vi "SessionManagerSimulator.vi"() -> ()   [LabVIEW 2014]
uses:
  TimeStamper/TimeStamper.lvclass
panel:
  out "error out":errorcluster
  in  "Experimenter":string(combo)="Unselected"
  out "Session Path":path
  in  "stop":bool
  in  "Subject":string(combo)="Testing"
  in  "Counter Card":tag="Dev1"
  in  "Sample Lines":tag[](array[tag])=["/Dev3/ai/StartTrigger", "/Dev1/PXI_Trig4", "/4498_1/ai/StartTrigger"]
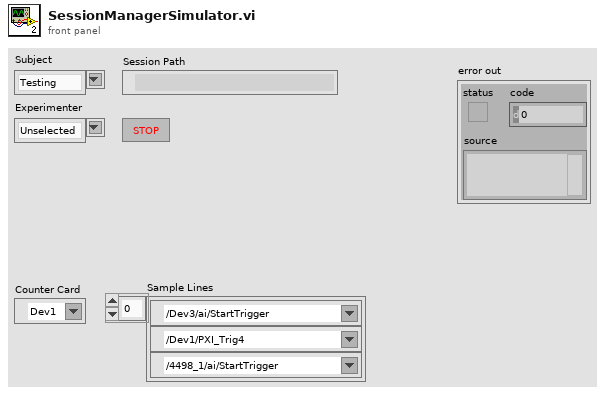
[diagram p1: front panel]
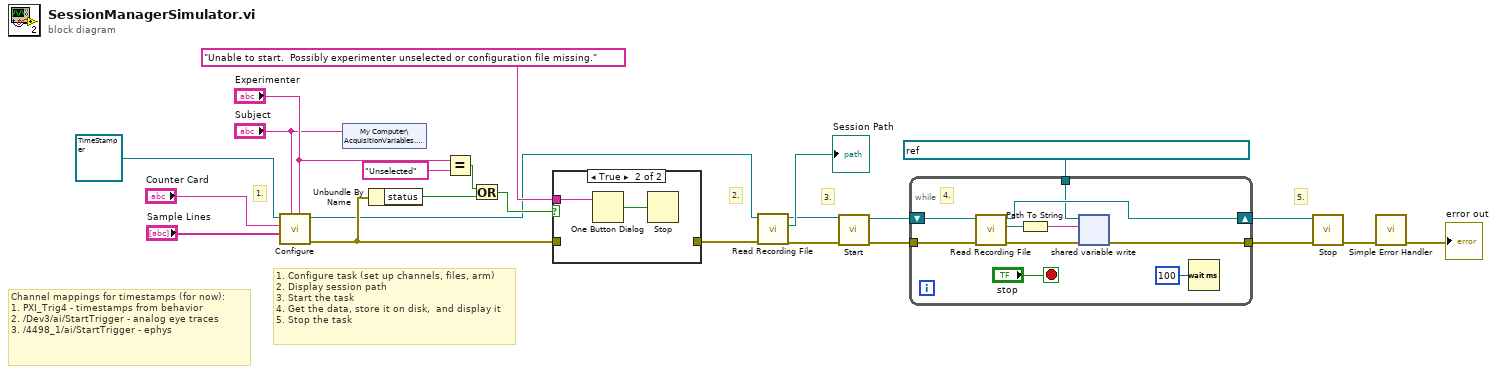
[diagram p0: block diagram]
diagram:
  # "Channel mappings for timestamps (for now):\n1. PXI_Trig4 - timestamps from behavior\n2. /Dev3/ai/StartTrigger - analog eye traces\n3. /4498_1/ai/StartTrigger - ephys"
  # "1. Configure task (set up channels, files, arm)\n2. Display session path\n3. Start the task\n4. Get the data, store it on disk,  and display it\n5. Stop the task"
  # "2."
  # "5."
  # "3."
  # "1."
  n1 = call-dynamic "Configure.vi"("Experimenter"="Experimenter", "Subject"="Subject", "Sample Lines"="Sample Lines", "DAQmx Device Name"="Counter Card", "TimeStamper in"=refnum<class "TimeStamper.lvclass"> refnum ("TimeStamper.lvclass")) -> ("error out"=w9:errorcluster, "TimeStamper out"=w8:refnum<class "TimeStamper.lvclass">)  [unwired: 5 in]
  n2 = shared-variable "My Computer\\AcquisitionVariables.lvlib\\Subject"("Subject") -> ()  [unwired: 1 in, 1 out]
  n3 = Unbundle By Name(w9) -> ("status"=w10:bool)
  n4 = Equal?(x="Experimenter", y="Unselected") -> (x = y?=w16:bool)
  n5 = Or(x=w16, y=w10) -> (x .or. y?=w15:bool)
  n6 = case shown="True" w15 {
    tunnel: "Unable to start.  Possibly experimenter unselected or configuration file missing." -> [_ w26]
    tunnel: w9 -> [w24 _]
    tunnel: [w24 _] -> w7
    frame False {
    }
    frame True {
      n7 = One Button Dialog(message=w26) -> (true=w25:bool)  [unwired: 1 in]
      n8 = Stop(stop? (T)=w25) -> ()
    }
  }
  n9 = call-dynamic "Read Recording File.vi"("error in (no error)"=w7, "AcquistionObject in"=w8) -> ("error out"=w4:errorcluster, "Recording File"=→"Session Path":path, "AcquistionObject out"=w5:refnum<class "TimeStamper.lvclass">)  [unwired: 7 in]
  n10 = call-dynamic "Start.vi"("error in (no error)"=w4, "TimeStamper in"=w5) -> ("error out"=w21:errorcluster, "TimeStamper out"=w20:refnum<class "TimeStamper.lvclass">)  [unwired: 8 in]
  n11 = while {
    tunnel: w21 -> [w31]
    shift-right: [w29] -> w19
    shift-left: w20 -> [w28]
    tunnel: [w30] -> w18
    tunnel: refnum<k21> "ni.var.psp://My Computer/AcquisitionVariables/SessionPath" ("shared variable refnum in") -> [w27]
    stop <- "stop" stop-if-true
    # "4."
    n12 = call-dynamic "Read Recording File.vi"("error in (no error)"=w31, "AcquistionObject in"=w28) -> ("error out"=w34:errorcluster, "Recording File"=w32:path, "AcquistionObject out"=w29:refnum<class "TimeStamper.lvclass">)  [unwired: 7 in]
    n13 = Path To String(path=w32) -> (string=w33:string)
    n14 = shared-variable-write(w27, w34, w33) -> (w30:errorcluster)  [unwired: 1 out]
    n15 = Wait (ms)(milliseconds to wait=u32 100) -> ()  [unwired: 1 out]
  }
  n16 = call-dynamic "Stop.vi"("error in (no error)"=w18, "TimeStamper in"=w19) -> ("error out"=w13:errorcluster)  [unwired: 8 in, 1 out]
  n17 = call <vilib>:"Simple Error Handler.vi"("error in (no error)"=w13) -> ("error out"=→"error out":errorcluster)  [unwired: 4 in, 4 out]
